vi "Check Raster Point In Range.vi"(11 "Projected Triangle":T1={"Vertex 1"={"Position"={"x"=0.0, "y"=0.0, "z"=0.0}, "UV"={"u"=0.0, "v"=0.0}, "Colour"=12517256}, "Vertex 2"={"Position"={"x"=0.0, "y"=0.0, "z"=0.0}, "UV"={"u"=0.0, "v"=0.0}, "Colour"=12517256}, "Vertex 3"={"Position"={"x"=0.0, "y"=0.0, "z"=0.0}, "UV"={"u"=0.0, "v"=0.0}, "Colour"=12517256}, "Colour"=0} {"Vertex 3"."UV"."v" min=0 max=1 step=0.1; "Vertex 3"."UV"."u" min=0 max=1 step=0.1; "Vertex 2"."UV"."v" min=0 max=1 step=0.1; "Vertex 2"."UV"."u" min=0 max=1 step=0.1; "Vertex 1"."UV"."v" min=0 max=1 step=0.1; "Vertex 1"."UV"."u" min=0 max=1 step=0.1}) -> (3 "Keep":bool)   [LabVIEW 2020, in "3D (FPGA).lvlib"]
uses:
  3D (FPGA).lvlib
  Raster/UV.ctl
  Raster/Raster (FPGA).lvlib
  Vector 3D.ctl
  Vertex.ctl
  Triangle.ctl
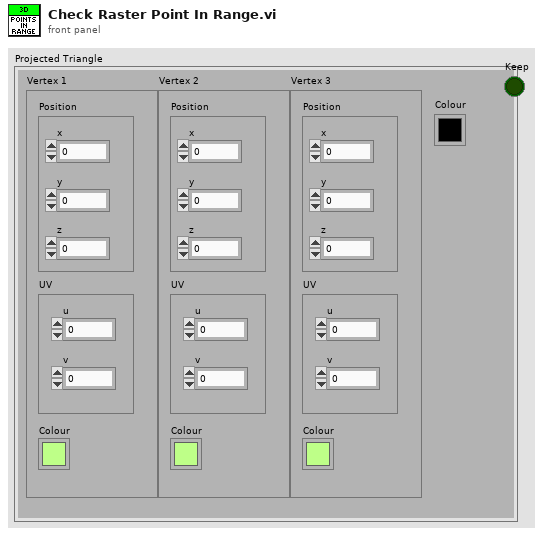
[diagram p1: front panel]
types:
  T1 = typedef "3D (FPGA).lvlib/Triangle.ctl" = cluster{"Vertex 1":T2, "Vertex 2":T2, "Vertex 3":T2, "Colour":u32}
  T2 = typedef "3D (FPGA).lvlib/Vertex.ctl" = cluster{"Position":T3, "UV":T4, "Colour":u32}
  T3 = typedef "3D (FPGA).lvlib/Vector 3D.ctl" = cluster{"x":sgl, "y":sgl, "z":sgl}
  T4 = typedef "Raster (FPGA).lvlib/UV.ctl" = cluster{"u":sgl, "v":sgl}
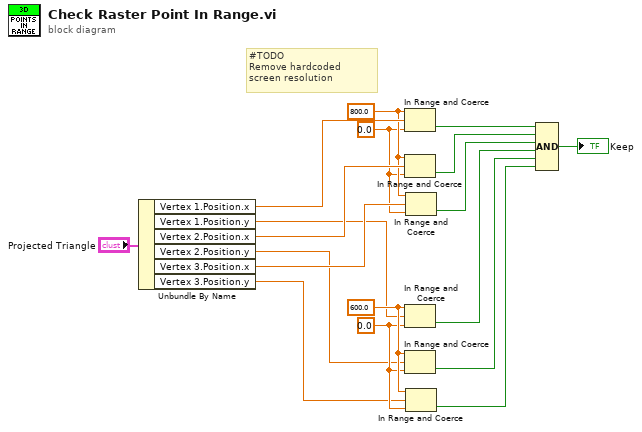
[diagram p0: block diagram]
diagram:
  w11 = sgl 0.0 ("lower limit")
  w12 = sgl 600.0 ("upper limit")
  w13 = sgl 0.0 ("lower limit")
  w14 = sgl 800.0 ("upper limit")
  # "#TODO\nRemove hardcoded screen resolution"
  n1 = Unbundle By Name("Projected Triangle") -> ("Vertex 1.Position.x"=w17:sgl, "Vertex 1.Position.y"=w10:sgl, "Vertex 2.Position.x"=w16:sgl, "Vertex 2.Position.y"=w9:sgl, "Vertex 3.Position.x"=w15:sgl, "Vertex 3.Position.y"=w8:sgl)
  n2 = In Range and Coerce(upper limit=w14, x=w17, lower limit=w13) -> (In Range?=w7:bool)  [unwired: 1 out]
  n3 = In Range and Coerce(upper limit=w14, x=w16, lower limit=w13) -> (In Range?=w6:bool)  [unwired: 1 out]
  n4 = In Range and Coerce(upper limit=w12, x=w10, lower limit=w11) -> (In Range?=w4:bool)  [unwired: 1 out]
  n5 = In Range and Coerce(upper limit=w12, x=w9, lower limit=w11) -> (In Range?=w3:bool)  [unwired: 1 out]
  n6 = In Range and Coerce(upper limit=w14, x=w15, lower limit=w13) -> (In Range?=w5:bool)  [unwired: 1 out]
  n7 = In Range and Coerce(upper limit=w12, x=w8, lower limit=w11) -> (In Range?=w2:bool)  [unwired: 1 out]
  n8 = Compound Arithmetic op=AND(w7, w6, w5, w4, w3, w2) -> (→"Keep":bool)
